vi "Vision Assistant1.vi"(0 "Color Plane (Color Plane Extraction 1)":i32(ring)=2 items=["Red", "Green", "Blue", "Hue", "Saturation", "Luminance", "Value", "Intensity"], 1 "Range (Threshold 1)":cluster{"Lower value":sgl, "Upper value":sgl}={"Lower value"=199.0, "Upper value"=255.0}, 2 "Number of Erosion (Adv. Morphology 1)":i32=1, 3 "Square/Hexa (Square) (Adv. Morphology 1)":bool, 4 "Connectivity 4/8 (8) (Adv. Morphology 1)":bool=TRUE, 5 "Low Pass/High Pass (Low) (Adv. Morphology 1)":bool, 7 "error in":errorcluster) -> (20 "Number of Matches (Shape Matching 1)":i32, 21 "Shape Report (calibrated) (Shape Matching 1)":T2(array[cluster]) {"Score" format="%.2f"; "Centroid"."y" format="%.2f"; "Centroid"."x" format="%.2f"}, 27 "error out":errorcluster)   [LabVIEW 2016]
uses:
  <vilib>/vision/driver/NI_Vision_Acquisition_Software.lvlib
  <vilib>/vision/NI_Vision_Development_Module.lvlib
panel:
  out "Image Out":T1(plugin-control)
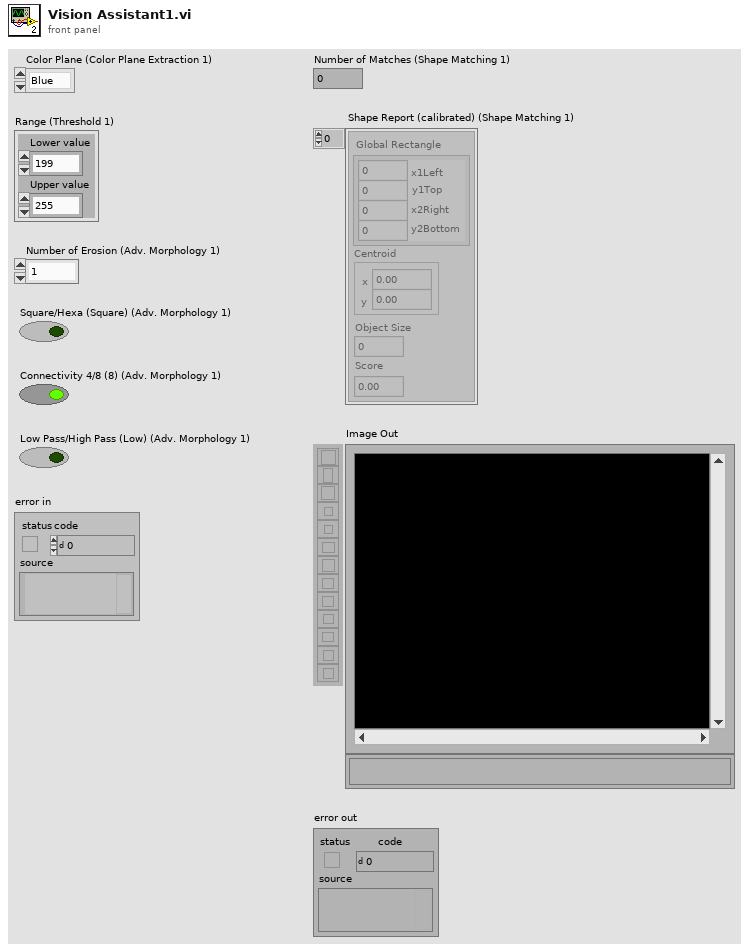
[diagram p1: front panel]
types:
  T1 = typedef "IMAQ Image.ctl" = refnum<image>
  T2 = cluster{"Global Rectangle":cluster{"x1Left":i32, "y1Top":i32, "x2Right":i32, "y2Bottom":i32}, "Centroid":cluster{"x":sgl, "y":sgl}, "Object Size":u32, "Score":dbl}[]
  T3 = typedef "IMAQdx.ctl" = refnum<k21>
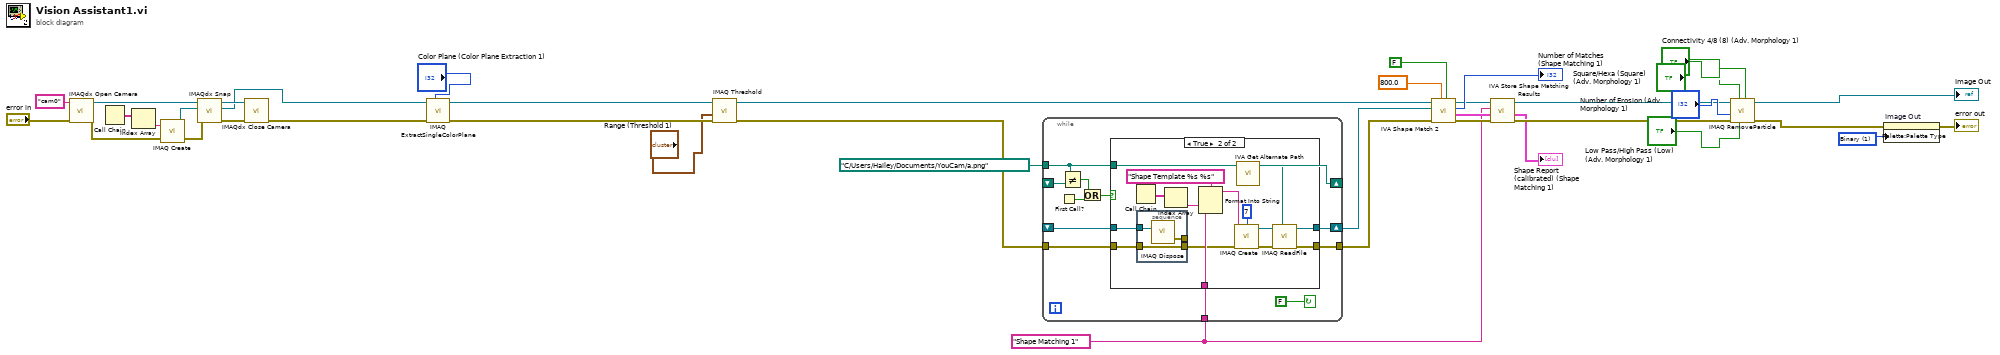
[diagram p0: block diagram]
diagram:
  w1 = u32 1 items=["Grayscale", "Binary", "Gradient", "Rainbow", "Temperature", "User Defined", "Binary 16 Bit", "Gradient 16 Bit", "Rainbow 16 Bit", "Temperature 16 Bit", "User Defined 16 Bit"] ("Palette Type")
  w10 = "Shape Matching 1" ("Step Name")
  n1 = call <vilib>:"IMAQdx Open Camera.vi"("error in"="error in", "Session In"="cam0" ("Interface Name")) -> ("error out"=w38:errorcluster, "Session Out"=w32:T3)  [unwired: 1 in, 7 out]
  n2 = Call Chain() -> (call chain=w30:string[])
  n3 = Index Array(array=w30) -> (element=w29:string)  [unwired: 1 in]
  n4 = call "IMAQ Create"("Image Name"=w29, "error in (no error)"=w38) -> ("New Image"=w34:T1, "error out"=w33:errorcluster)  [unwired: 2 in, 1 out]
  n5 = call <vilib>:"IMAQdx Snap.vi"("error in"=w33, "Image In"=w34, "Session In"=w32) -> ("error out"=w36:errorcluster, "Image Out"=w27:T1, "Session Out"=w37:T3)  [unwired: 6 out]
  n6 = call <vilib>:"IMAQdx Close Camera.vi"("error in"=w36, "Session In"=w37) -> ("error out"=w35:errorcluster)  [unwired: 9 out]
  n7 = call "IMAQ ExtractSingleColorPlane"("Color Plane"="Color Plane (Color Plane Extraction 1)", "error in (no error)"=w35, "Image Src"=w27) -> ("error out"=w26:errorcluster, "Image Dst Out"=w24:T1)  [unwired: 1 in, 6 out]
  n8 = call "IMAQ Threshold"("error in (no error)"=w26, "Range"="Range (Threshold 1)", "Image Src"=w24) -> ("error out"=w23:errorcluster, "Image Dst Out"=w19:T1)  [unwired: 3 in, 4 out]
  n9 = while {
    shift-right: [w50] -> w11
    shift-left: _ -> [w49]
    tunnel: [w47] -> w12
    tunnel: w23 -> [w46]
    tunnel: path "C:/Users/Hailey/Documents/YouCam/a.png" ("Template Path") -> [w44]
    tunnel: w10 -> [w45]
    shift-right: [w44] -> _
    shift-left: _ -> [w43]
    stop <- FALSE continue-if-true
    n10 = First Call?() -> (First Call?: T/F=w42:bool)
    n11 = Not Equal?(x=w44, y=w43) -> (x != y?=w41:bool)
    n12 = Or(x=w41, y=w42) -> (x .or. y?=w40:bool)
    n13 = case shown="True" w40 {
      tunnel: [w52 w64] -> w50
      tunnel: w49 -> [w52 w55]
      tunnel: [w51 w62] -> w47
      tunnel: w46 -> [w51 w54]
      tunnel: w44 -> [_ w57]
      tunnel: w45 -> [_ w58]
      frame False {
      }
      frame True {
        n14 = Call Chain() -> (call chain=w60:string[])
        n15 = stacked-sequence {
          tunnel: w55 -> [w70]
          tunnel: w54 -> [w69]
          tunnel: [w69] -> w53
          tunnel: [w68] -> _
          frame #0 {
            n16 = call "IMAQ Dispose"("Image"=w70) -> ("error out"=w68:errorcluster)  [unwired: 2 in, 3 out]
          }
        }
        n17 = Index Array(array=w60) -> (element=w59:string)  [unwired: 1 in]
        n18 = Format Into String(format string="Shape Template %s %s" ("Image Name"), w59, w58) -> (resulting string=w67:string)  [unwired: 2 in, 1 out]
        n19 = call "IMAQ Create"("Border Size"=7, "Image Name"=w67, "error in (no error)"=w53) -> ("New Image"=w65:T1, "error out"=w63:errorcluster)  [unwired: 1 in, 1 out]
        n20 = call <vilib>:"IVA Get Alternate Path.vi"("Path In"=w57) -> ("Path Out"=w56:path)  [unwired: 10 out]
        n21 = call "IMAQ ReadFile"("File Path"=w56, "error in (no error)"=w63, "Image"=w65) -> ("error out"=w62:errorcluster, "Image Out"=w64:T1)  [unwired: 2 in, 5 out]
      }
    }
  }
  n22 = call <vilib>:"IVA Shape Match 2.vi"("Scale Invariance"=FALSE, "Minimal Score"=800.0, "error in (no error)"=w12, "Template"=w11, "Image Src"=w19) -> ("error out"=w18:errorcluster, "Shape Report"=w16:T2, "Number of Matches"=→"Number of Matches (Shape Matching 1)":i32, "Image Out"=w15:T1)  [unwired: 3 out]
  n23 = call <vilib>:"IVA Store Shape Matching Results.vi"("error in (no error)"=w18, "Shape Report"=w16, "Step Name"=w10, "Image in"=w15) -> ("error out"=w17:errorcluster, "Shape Report (calibrated)"=→"Shape Report (calibrated) (Shape Matching 1)":T2, "Image dup"=w5:T1)  [unwired: 5 out]
  n24 = call "IMAQ RemoveParticle"("Connectivity 4/8 (8)"="Connectivity 4/8 (8) (Adv. Morphology 1)", "Low Pass/High Pass (Low)"="Low Pass/High Pass (Low) (Adv. Morphology 1)", "Square/Hexa (Square)"="Square/Hexa (Square) (Adv. Morphology 1)", "error in (no error)"=w17, "Number of Erosion"="Number of Erosion (Adv. Morphology 1)", "Image Src"=w5) -> ("error out"=w4:errorcluster, "Image Dst Out"=→"Image Out":T1)  [unwired: 1 in, 3 out]
  n25 = property on="Image Out" class="ImageControl"(error in=w4, "Palette:Palette Type"=w1) -> (error out=→"error out":errorcluster)  [unwired: 1 in, 1 out]
